vi "LIA_FPGA4a1.vi"(0 "nominal freq":fxp<+,16,0>=0.010009765625, 1 "dec1":i16=1, 3 "stages":i8=1, 11 "K":fxp<+,16,0>=0.001007080078125, 12 "dec2":i16=1, 14 "decimation":i16=1024, 15 "While Loop Counter":i32) -> (4 "channelI":i64, 5 "Nominal Freq":fxp<+/-,64,32>, 6 "channelQ":i64, 9 "K Constant":fxp<+/-,32,16>, 13 "f":fxp<+/-,32,0> format="%.32g")   [LabVIEW 2012]
uses:
  <vilib>/rvi/DataTransferAndStorage/Container/Common/niFpgaContainerMetaDataKey.ctl
  <vilib>/rvi/DataTransferAndStorage/Container/Common/niFpgaContainerState.ctl
  <vilib>/rvi/DataTransferAndStorage/Container/Common/niFpgaDataTypeControl.ctl
  <vilib>/rvi/DataTransferAndStorage/Container/Common/niFpgaContainerImplementationControl.ctl
  <vilib>/rvi/DataTransferAndStorage/Container/Common/niFpgaContainerArbitrationOptionsControl.ctl
  <vilib>/rvi/DataTransferAndStorage/Container/Common/niFpgaTransferTypeControl.ctl
  <vilib>/rvi/DataTransferAndStorage/Container/Common/niFpgaContainerInitializationParameters.ctl
  <vilib>/rvi/Memory/Memory_Types/niFpgaMemoryInterfaceConfiguration.ctl
  <vilib>/rvi/FIFO/Fifo_Types/niFpgaFifoControlLogicControl.ctl
  <vilib>/rvi/DataTransferAndStorage/Container/Common/niFpgaContainerGetUniqueNameForEmu.vi
  <vilib>/rvi/DataTransferAndStorage/Container/Common/niFpgaContainerSetEmuInfo.vi
  <vilib>/rvi/eio/common/nirviEmuReportErrorAndStop.vi
  <vilib>/rvi/eio/common/nirviEmuTemplateMethod_errors.vi
  <vilib>/rvi/Emulation/niFpgaSctlEmulationGetInTimedLoop.vi
  <vilib>/rvi/FIFO/Fifo_Resource/nirvififoEmulationSetSize.vi
  <vilib>/rvi/Emulation/niFpgaSctlEmulationFifoFullMgr.vi
  <vilib>/rvi/errors/niFpgaSetErrorForExecOnDevCompSimple.vi
  <vilib>/rvi/Emulation/niFpgaSctlEmulationResourceMgr.vi
  <vilib>/rvi/LocalResourceManager/LocalResourceManager.xnode
  <vilib>/rvi/FXPMathLib/FxpInterpret/XNode/nifxpmath_Interpret.xnode
  <vilib>/eio/EIONode/EIONode.xnode
  <vilib>/rvi/DataTransferAndStorage/Container/XNode/niFpgaContainer.xnode
  <vilib>/rvi/FIFO/Fifo_Resource/nirvififoEmulationRead.vi
  <vilib>/rvi/FIFO/Fifo_Resource/nirvififoEmulationWrite.vi
panel:
  out "ref":i16 format="%.0x"
  out "sig":i16 format="%.0x"
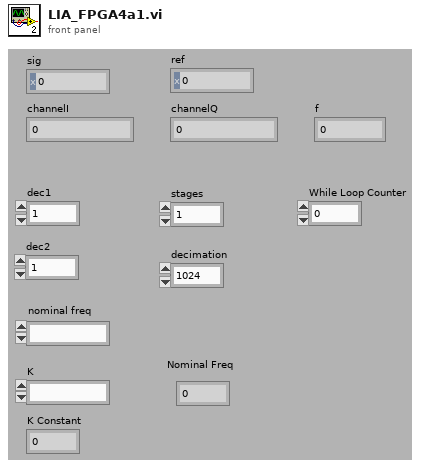
[diagram p1: front panel]
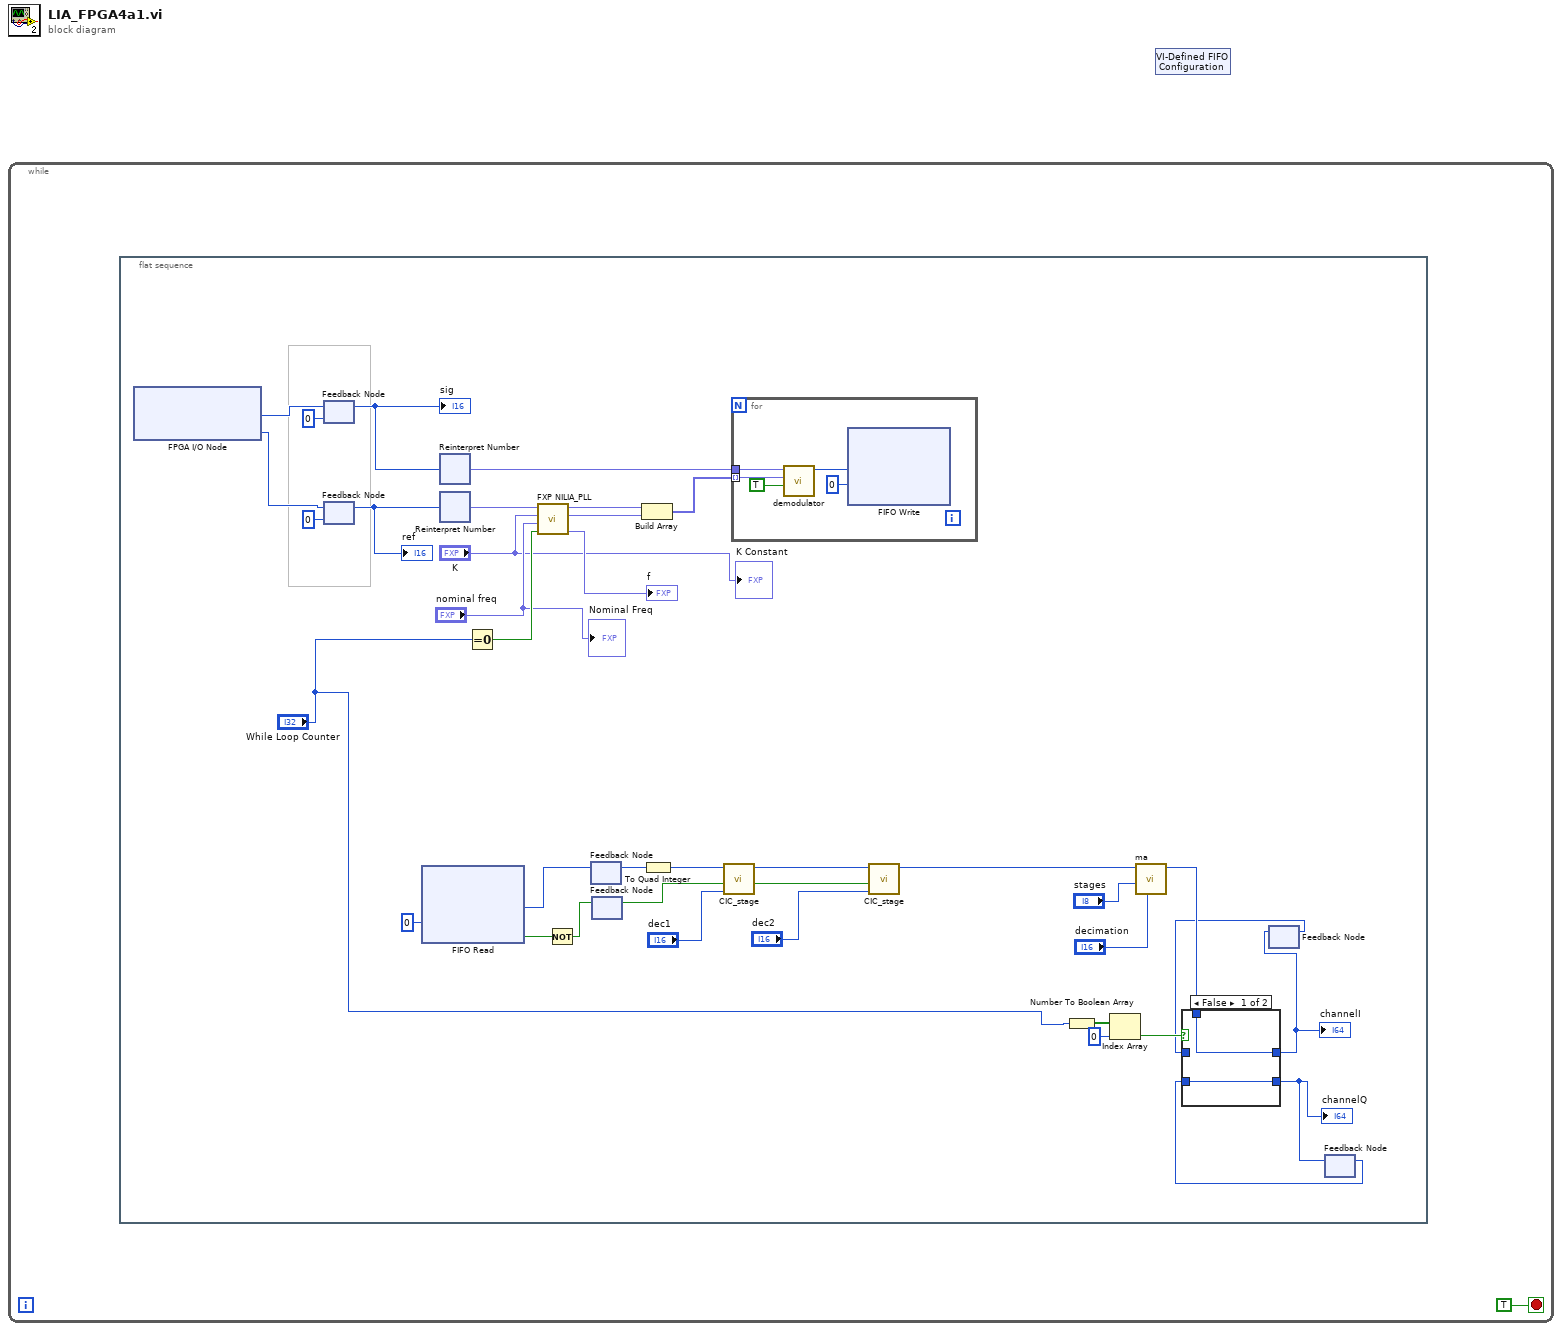
[diagram p0: block diagram]
diagram:
  n1 = while {
    stop <- TRUE stop-if-true
    n2 = flat-sequence {
      frame #0 {
        n3 = xnode "FPGA I/O Node"() -> ("Connector0/AI7"=w35:i16, "Connector0/AI6"=w2:i16)  [unwired: 2 in, 2 out]
        n4 = feedback #1(i16 0 ("y")) -> (w34:i16)
        "sig" <- w34
        n5 = feedback-in #1(w35) -> ()
        n6 = feedback #2(i16 0 ("z [I32.1]")) -> (w33:i16)
        "ref" <- w33
        n7 = feedback-in #2(w2) -> ()
        n8 = xnode ("FIFO Read")("Timeout"=0) -> ("Element"=w12:i32, "Timed Out?"=w11:bool)  [unwired: 1 in, 1 out]
        n9 = xnode "Reinterpret Number"("x"=w34) -> ("y"=w38:fxp<+/-,16,1>)
        n10 = xnode "Reinterpret Number"("x"=w33) -> ("y"=w32:fxp<+/-,16,1>)
        n11 = Equal To 0?(x="While Loop Counter") -> (x = 0?=w28:bool)
        n12 = call "FXP NILIA_PLL.vi"("reset?"=w28, "norminal freq [U16.0]"="nominal freq", "alpha [U16.0]"="K", "x[I16.1]"=w32) -> ("f"=→"f":fxp<+/-,32,0>, "sin(z)"=w30:fxp<+/-,16,2>, "cos(z)"=w29:fxp<+/-,16,2>)  [unwired: 4 in, 1 out]
        n13 = Not(x=w11) -> (.not. x?=w10:bool)
        n14 = feedback #3() -> (w14:i32)  [unwired: 1 out]
        n15 = feedback-in #3(w12) -> ()
        n16 = feedback #4() -> (w8:bool)  [unwired: 1 out]
        n17 = feedback-in #4(w10) -> ()
        n18 = Build Array(w29, w30) -> (w39:fxp<+/-,16,2>[])
        n19 = To Quad Integer(1:w14) -> (0:w9:i64)
        n20 = call "CIC_stage.vi"("decimate factor"="dec1", "New Data"=w8, "input"=w9) -> ("Data Ready"=w6:bool, "output"=w7:i64)  [unwired: 7 out]
        n21 = for {
          tunnel: w38 -> [w46]
          tunnel: w39 -> [w44] mode=indexing
          n22 = call "demodulator.vi"("New Data"=TRUE, "ref"=w44, "signal"=w46) -> ("x*y"=w47:i32)  [unwired: 8 out]
          n23 = xnode ("FIFO Write")("Element"=w47, "Timeout"=0) -> ()  [unwired: 1 in, 2 out]
        }
        n24 = call "CIC_stage.vi"("decimate factor"="dec2", "New Data"=w6, "input"=w7) -> ("output"=w23:i64)  [unwired: 8 out]
        n25 = Number To Boolean Array(number="While Loop Counter") -> (Boolean array=w22:bool[])
        n26 = Index Array "Index Array"(array=w22, index=0) -> (element=w20:bool)
        n27 = call "ma.vi"("decimate"="decimation", "stages"="stages", "input"=w23) -> ("output"=w19:i64)  [unwired: 8 out]
        n28 = feedback #5() -> (w17:i64)  [unwired: 1 in]
        n29 = feedback #6() -> (w15:i64)  [unwired: 1 in]
        n30 = case shown="False" w20 {
          tunnel: w19 -> [w41 w43]
          tunnel: [w41 w42] -> w18
          tunnel: [w40 w43] -> w16
          tunnel: w17 -> [_ w42]
          tunnel: w15 -> [w40 _]
          frame False {
          }
          frame True {
          }
        }
        "channelI" <- w18
        "channelQ" <- w16
        n31 = feedback-in #5(w18) -> ()
        n32 = feedback-in #6(w16) -> ()
        "Nominal Freq" <- "nominal freq"
        "K Constant" <- "K"
      }
    }
  }
  n33 = xnode "VI-Defined FIFO Configuration"() -> ()  [unwired: 1 out]
